vi "recoreder.vi"() -> ()   [LabVIEW 2018]
uses:
  <vilib>/sound2/lvsound2.llb/Sound Data Format.ctl
  <vilib>/sound2/lvsound2.llb/Sound File Write Open.vi
  <vilib>/sound2/lvsound2.llb/Sound File Write (DBL).vi
panel:
  in  "sound format":T1={"sample rate (S/s)"=22050.0, "number of channels"=2, "bits per sample"=16}
  in  "path":path
  out "Data":dynamicdata(graph)
  in  "Record Time":dbl
  in  "Device(Default: 0)":u32 caption="Device"
  in  "Start":bool
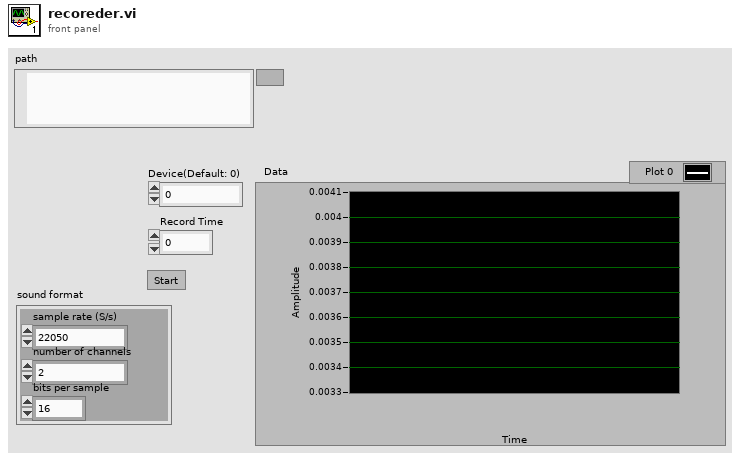
[diagram p1: front panel]
types:
  T1 = typedef "Sound Data Format.ctl" = cluster{"sample rate (S/s)":dbl, "number of channels":i32, "bits per sample":i32}
  T2 = typedef "Sound File Refnum.ctl" = refnum<file>
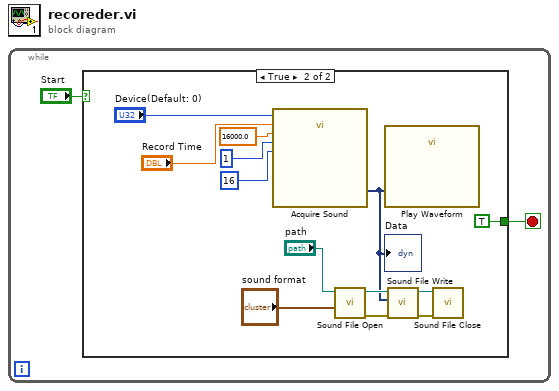
[diagram p0: block diagram]
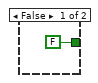
[diagram p2: hidden frame]
diagram:
  n1 = while {
    stop <- w1 stop-if-true
    n2 = case shown="True" "Start" {
      tunnel: [FALSE TRUE] -> w1
      frame False {
      }
      frame True {
        n3 = call "Acquire Sound"("Device"="Device(Default: 0)", "Duration (s)"="Record Time", "Sample rate (Hz)"=16000.0, "#Channels"=1, "Resolution (bits)"=16) -> ("Data"=w4:dynamicdata)  [unwired: 13 in, 1 out]
        "Data" <- w4
        n4 = call-poly <vilib>:"Sound File Open.vi"("sound format"="sound format", "path"="path") -> ("error out"=w8:errorcluster, "sound file refnum"=w9:T2)  [unwired: 8 in]
        n5 = call "Play Waveform"("Data"=w4) -> ()  [unwired: 18 in, 1 out]
        n6 = call-poly <vilib>:"Sound File Write.vi"("error in (no error)"=w8, "data"=w4, "sound file refnum"=w9) -> ("error out"=w6:errorcluster, "sound file refnum out"=w7:T2)  [unwired: 7 in]
        n7 = call <vilib>:"Sound File Close.vi"("error in (no error)"=w6, "sound file refnum"=w7) -> ()  [unwired: 9 in, 1 out]
      }
    }
  }
